vi "TDC_getTimebase.vi"(8 "Error In":errorcluster) -> (0 "Error Out":errorcluster, 3 "Time Base [s]":dbl)   [LabVIEW 2011]
uses:
  tdcbase.dll
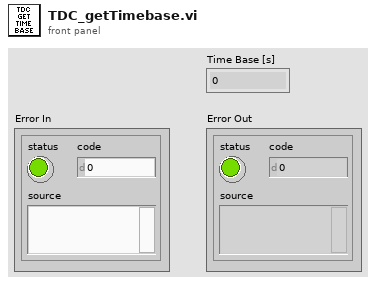
[diagram p1: front panel]
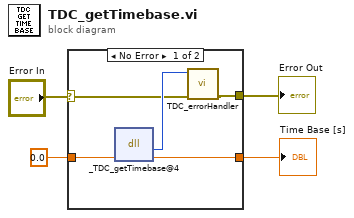
[diagram p0: block diagram]
diagram:
  n1 = case shown="No Error" "Error In" {
    selector: "Error In" -> [w5 w10]
    tunnel: [w8 w10] -> w4
    tunnel: [w7 w11] -> w3
    tunnel: 0.0 -> [w6 w11]
    frame No Error {
      n2 = dll-call lib="X:/tdcbase.dll" fn="_TDC_getTimebase@4"("timebase"=w6) -> ("return type"=w9:i32, "timebase"=w7:dbl)  [unwired: 3 in, 2 out]
      n3 = call "TDC_errorHandler.vi"("Error In"=w5, "TDC Return Code"=w9) -> ("Error Out"=w8:errorcluster)  [unwired: 9 in]
    }
    frame Error {
    }
  }
  "Time Base [s]" <- w3
  "Error Out" <- w4
